vi "Calculate String Checksum.vi"(11 "String":string) -> (3 "Checksum":u8 format="0x%02x")   [LabVIEW 2020, in "nmea.lvlib" / "NMEA Message.lvclass"]
uses:
  NMEA Message.lvclass
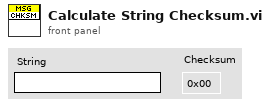
[diagram p1: front panel]
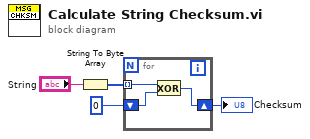
[diagram p0: block diagram]
diagram:
  n1 = String To Byte Array(string="String") -> (unsigned byte array=w3:u8[])
  n2 = for {
    tunnel: w3 -> [w7] mode=indexing
    shift-right: [w5] -> w1
    shift-left: u8 0 -> [w6]
    n3 = Exclusive Or(1:w6, 2:w7) -> (0:w5:u8)
  }
  "Checksum" <- w1
